vi "example_GTimeout.vi"() -> ()   [LabVIEW 2021]
uses:
  <vilib>/Galil/resources/gclib/gclib.lvlib
  <vilib>/Galil/resources/gclibo/gclibo.lvlib
panel:
  out "Interrupt":u8
  out "Error Out":errorcluster
  in  "timeout_ms":i16=1000
  in  "IP Address":string="192.168.1.77 -s EI"
  in  "Command":string="EI1; SHA; PA 5000; BGA"
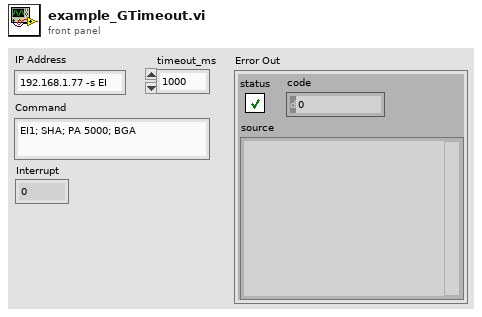
[diagram p1: front panel]
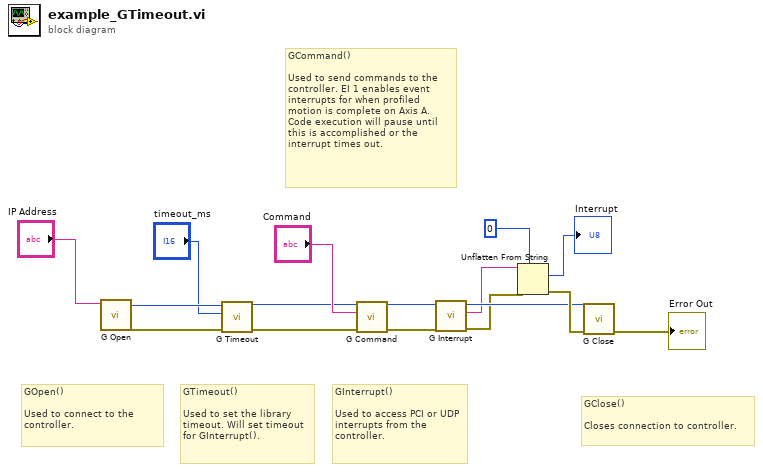
[diagram p0: block diagram]
diagram:
  # "GClose()\n\nCloses connection to controller."
  # "GTimeout()\n\nUsed to set the library timeout. Will set timeout for GInterrupt()."
  # "GInterrupt()\n\nUsed to access PCI or UDP interrupts from the controller."
  # "GCommand()\n\nUsed to send commands to the controller. EI 1 enables event interrupts for when profiled motion is complete on Axis A. Code execution will pause until this is accomplished or the interrupt times out."
  # "GOpen()\n\nUsed to connect to the controller."
  n1 = call <vilib>:"G Open.vi"("address"="IP Address") -> ("error out"=w12:errorcluster, "g out"=w9:u64)  [unwired: 8 in]
  n2 = call <vilib>:"G Timeout.vi"("error in (no error)"=w12, "timeout_ms"="timeout_ms", "g"=w9) -> ("error out"=w11:errorcluster, "g out"=w10:u64)  [unwired: 6 in]
  n3 = call <vilib>:"G Command.vi"("g"=w10, "command"="Command", "error in (no error)"=w11) -> ("g out"=w14:u64, "error out"=w13:errorcluster)  [unwired: 10 in, 1 out]
  n4 = call <vilib>:"G Interrupt.vi"("error in (no error)"=w13, "g"=w14) -> ("error out"=w3:errorcluster, "status_byte out"=w2:string, "g out"=w4:u64)  [unwired: 7 in]
  n5 = Unflatten From String(type=u8 0, binary string=w2, error in (no error)=w3) -> (value=→"Interrupt":u8, error out=w6:errorcluster)  [unwired: 2 in, 1 out]
  n6 = call <vilib>:"G Close.vi"("error in (no error)"=w6, "g"=w4) -> ("error out"=→"Error Out":errorcluster)  [unwired: 9 in]
